vi "Point_string_to_points.vi"(4 "Points String":string) -> (1 "Points":cluster{"X":sgl, "Y":sgl}[](array[cluster]), 2 "Num Points":i32)   [LabVIEW 2018]
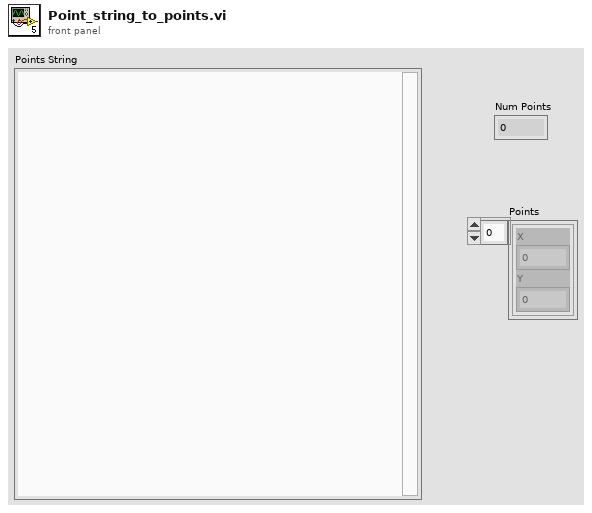
[diagram p1: front panel]
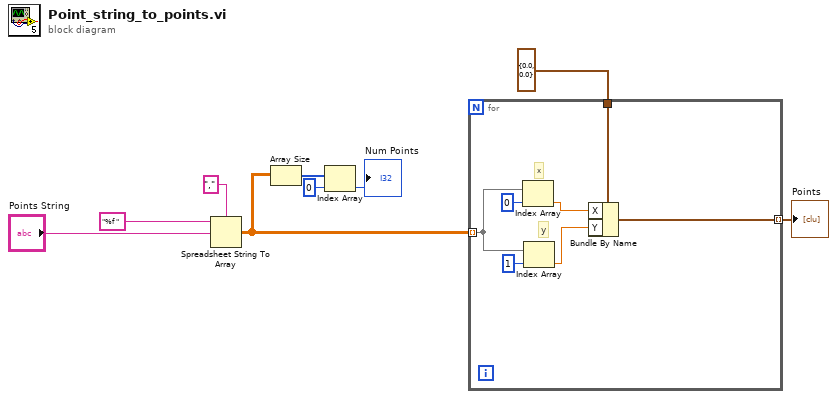
[diagram p0: block diagram]
diagram:
  n1 = Spreadsheet String To Array(delimiter (Tab)=",", format string="%f ", spreadsheet string="Points String") -> (array=w4:dbl[][])  [unwired: 1 in]
  n2 = Array Size(array=w4) -> (size(s)=w3:i32[])
  n3 = Index Array(array=w3, index=0) -> (element=→"Num Points":i32)
  n4 = for {
    tunnel: w4 -> [w16] mode=indexing
    tunnel: cluster{"X":sgl, "Y":sgl} {"X"=0.0, "Y"=0.0} ("Pixel pos") -> [w13]
    tunnel: [w10] -> w8 mode=indexing
    # "y"
    # "x"
    n5 = Index Array(array=w16, index=0) -> (element=w12:dbl)
    n6 = Index Array(array=w16, index=1) -> (element=w11:dbl)
    n7 = Bundle By Name(cluster=w13, "X"=w12, "Y"=w11) -> (w10:cluster{"X":sgl, "Y":sgl})
  }
  "Points" <- w8
